vi "MatlabGlobals.vi"() -> ()   [LabVIEW 2017]
panel:
  out "MatlabGlobalControlUpdateByNameCollection":variant
  out "MatlabGlobalControlRefBindingByExperiment":variant
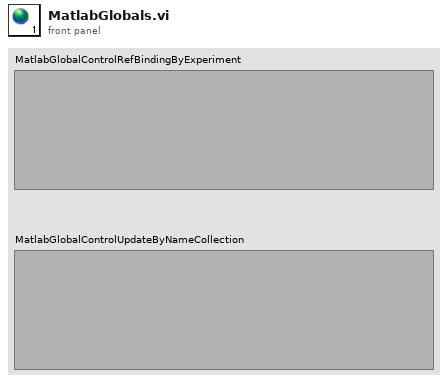
[diagram p1: front panel]
diagram:
